vi "Replace Array Element.vi"(4 "Replacement":string, 5 "Key name":string, 6 "Index":i32=4, 7 "Section name":string, 8 "error in (no error)":errorcluster, 9 "Use Key Regex? [F]":bool, 10 "Use Section Regex? [F]":bool, 11 "Carya Config in":refnum<class "Carya Config.lvclass">) -> (0 "error out":errorcluster, 3 "Carya Config out":refnum<class "Carya Config.lvclass">)   [LabVIEW 2013, in "Carya Config.lvclass"]
doc: "Copyright 2018, Carya Automatisering, Wiebe Walstra."
uses:
  Carya Config.lvclass
  CConfig Object/Search Replace Query/Search Replace Query.lvclass
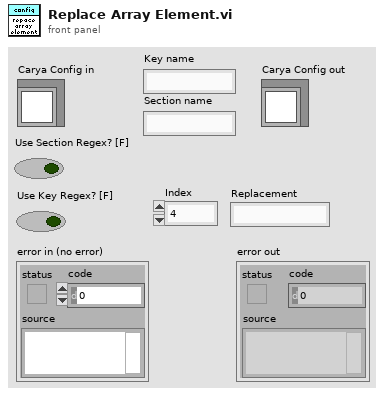
[diagram p1: front panel]
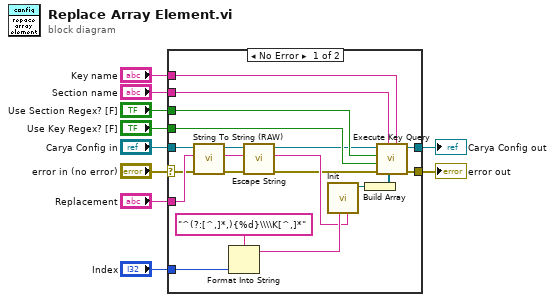
[diagram p0: block diagram]
diagram:
  n1 = case shown="No Error" "error in (no error)" {
    selector: "error in (no error)" -> [w11 w32]
    tunnel: [w30 w32] -> w9
    tunnel: [w29 w31] -> w7
    tunnel: "Carya Config in" -> [w15 w31]
    tunnel: "Section name" -> [w26 _]
    tunnel: "Key name" -> [w25 _]
    tunnel: "Use Section Regex? [F]" -> [w28 _]
    tunnel: "Use Key Regex? [F]" -> [w27 _]
    tunnel: "Index" -> [w20 _]
    tunnel: "Replacement" -> [w24 _]
    frame No Error {
      n2 = call-dynamic "String To String (RAW).vi"("error in (no error)"=w11, "String"=w24, "Registry Object"=w15) -> ("error out"=w13:errorcluster, "String (RAW)"=w17:string, "Registry Object"=w16:refnum<class "Carya Config.lvclass">)  [unwired: 6 in]
      n3 = Format Into String(format string="^(?:[^,]*,){%d}\\\\K[^,]*" ("Regex"), w20) -> (resulting string=w19:string)  [unwired: 2 in, 1 out]
      n4 = call-dynamic "Escape String.vi"("error in (no error)"=w13, "String"=w17, "Registry Object"=w16) -> ("error out"=w12:errorcluster, "Escaped string"=w18:string, "Registry Object"=w14:refnum<class "Carya Config.lvclass">)  [unwired: 6 in]
      n5 = call "Init.vi"("Replace"=w18, "Search"=w19) -> ("Find First Query out"=w23:refnum<class "Search Replace Query.lvclass">)  [unwired: 8 in, 1 out]
      n6 = Build Array(w23) -> (w22:refnum<class "Search Replace Query.lvclass">[])
      n7 = call-dynamic "Execute Key Query.vi"("Key name"=w25, "Key queries"=w22, "Section name"=w26, "error in (no error)"=w12, "Use Key Regex? [F]"=w27, "Use Section Regex? [F]"=w28, "Carya Config in"=w14) -> ("error out"=w30:errorcluster, "Carya Config out"=w29:refnum<class "Carya Config.lvclass">)  [unwired: 2 in, 1 out]
    }
    frame Error {
    }
  }
  "error out" <- w9
  "Carya Config out" <- w7
